vi "Get Symbol Information.vi"(8 "error in (no error)":errorcluster, 10 "Name":string, 11 "TwinCAT ADS in":refnum<class "TwinCAT ADS.lvclass">) -> (0 "error out":errorcluster, 1 "Symbol Info":refnum<k24>, 3 "TwinCAT ADS out":refnum<class "TwinCAT ADS.lvclass">)   [LabVIEW 2018, in "TwinCAT ADS.lvclass"]
uses:
  TwinCAT ADS.lvclass
  TwinCAT.Ads
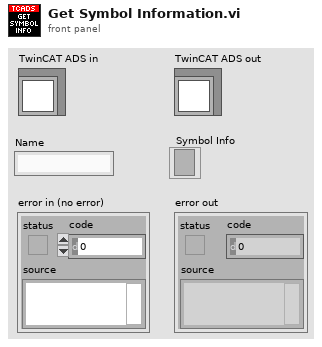
[diagram p1: front panel]
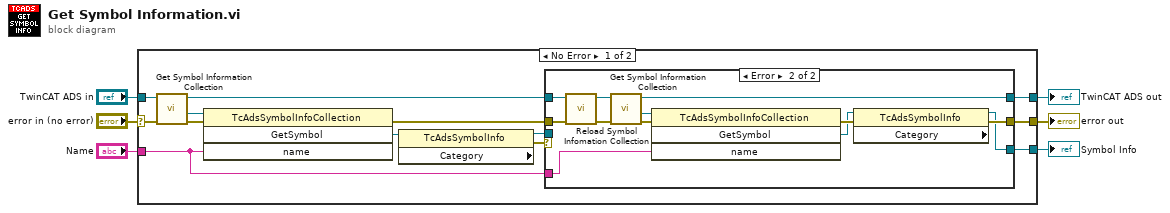
[diagram p0: block diagram]
diagram:
  n1 = case shown="No Error" "error in (no error)" {
    selector: "error in (no error)" -> [w18 w36]
    tunnel: [w9 w36] -> w2
    tunnel: [w10 w35] -> w4
    tunnel: "TwinCAT ADS in" -> [w19 w35]
    tunnel: "Name" -> [w7 _]
    tunnel: [w8 _] -> w1
    frame No Error {
      n2 = call-dynamic "Get Symbol Information Collection.vi"("error in (no error)"=w18, "TwinCAT ADS in"=w19) -> ("error out"=w17:errorcluster, "Symbol Info Collection"=w16:refnum<k24>, "TwinCAT ADS out"=w12:refnum<class "TwinCAT ADS.lvclass">)  [unwired: 7 in]
      n3 = invoke class="TcAdsSymbolInfoCollection" method="GetSymbol"(reference=w16, error in=w17, "name"=w7) -> (error out=w13:errorcluster, "GetSymbol"=w15:refnum<k24>)  [unwired: 1 in, 2 out]
      n4 = property class="TcAdsSymbolInfo" props=["Category"](reference=w15) -> (reference out=w11:refnum<k24>, error out=w14:errorcluster)  [unwired: 1 in, 1 out]
      n5 = case shown="Error" w14 {
        tunnel: w13 -> [w21 w34]
        tunnel: w12 -> [w20 w33]
        tunnel: [w21 w26] -> w9
        tunnel: [w20 w25] -> w10
        tunnel: [w22 w24] -> w8
        tunnel: w11 -> [w22 _]
        tunnel: w7 -> [_ w23]
        frame No Error {
        }
        frame Error {
          n6 = call-dynamic "Reload Symbol Infomation Collection.vi"("error in (no error)"=w34, "TwinCAT ADS in"=w33) -> ("error out"=w32:errorcluster, "TwinCAT ADS out"=w31:refnum<class "TwinCAT ADS.lvclass">)  [unwired: 8 in]
          n7 = call-dynamic "Get Symbol Information Collection.vi"("error in (no error)"=w32, "TwinCAT ADS in"=w31) -> ("error out"=w30:errorcluster, "Symbol Info Collection"=w29:refnum<k24>, "TwinCAT ADS out"=w25:refnum<class "TwinCAT ADS.lvclass">)  [unwired: 7 in]
          n8 = invoke class="TcAdsSymbolInfoCollection" method="GetSymbol"(reference=w29, error in=w30, "name"=w23) -> (error out=w28:errorcluster, "GetSymbol"=w27:refnum<k24>)  [unwired: 1 in, 2 out]
          n9 = property class="TcAdsSymbolInfo" props=["Category"](reference=w27, error in=w28) -> (reference out=w24:refnum<k24>, error out=w26:errorcluster)  [unwired: 1 out]
        }
      }
    }
    frame Error {
    }
  }
  "error out" <- w2
  "TwinCAT ADS out" <- w4
  "Symbol Info" <- w1
